vi "PumpValve3.vi"() -> ()   [LabVIEW 2015]
uses:
  PumpValve.ctl
  <vilib>/DAQmx/write.llb/DAQmx Write (Digital 1D Bool NChan 1Samp 1Line).vi
  <vilib>/DAQmx/miscellaneous.llb/DAQmx Fill In Error Info.vi
panel:
  in  "DAQmx Task 3":refnum<k21>
  in  "DAQmx Task 2":refnum<k21>
  in  "DAQmx Task 1":refnum<k21>
  in  "On/Off (Pump)":bool
  in  "Open/Close (Blue)":bool
  in  "Open/Close (Green)":bool
  in  "Manual Mode":bool
  in  "Stop Pumps/Valve":bool
  out "Invalid fill%":bool
  out "Tank":u32(slide) scale=0.0..100.0
  in  "Drain %":u32
  in  "Fill %":u32
  in  "Drain":bool
  in  "Stop Program":bool
  in  "Fill":bool
  out "Green":i32
  out "Blue":i32
  out "Pump":i32
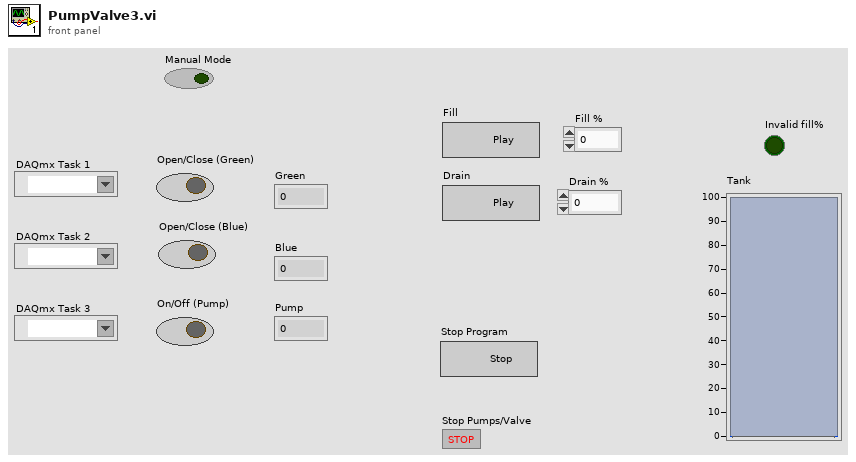
[diagram p1: front panel]
types:
  T1 = typedef "PumpValve.ctl" = enum16{"Manual", "Initialize", "Idle", "Fill", "Drain", "Stop"}
  T2 = cluster{"Open/Close (Green)":bool, "Open/Close (Blue)":bool, "On/Off (Pump)":bool, "off":bool}
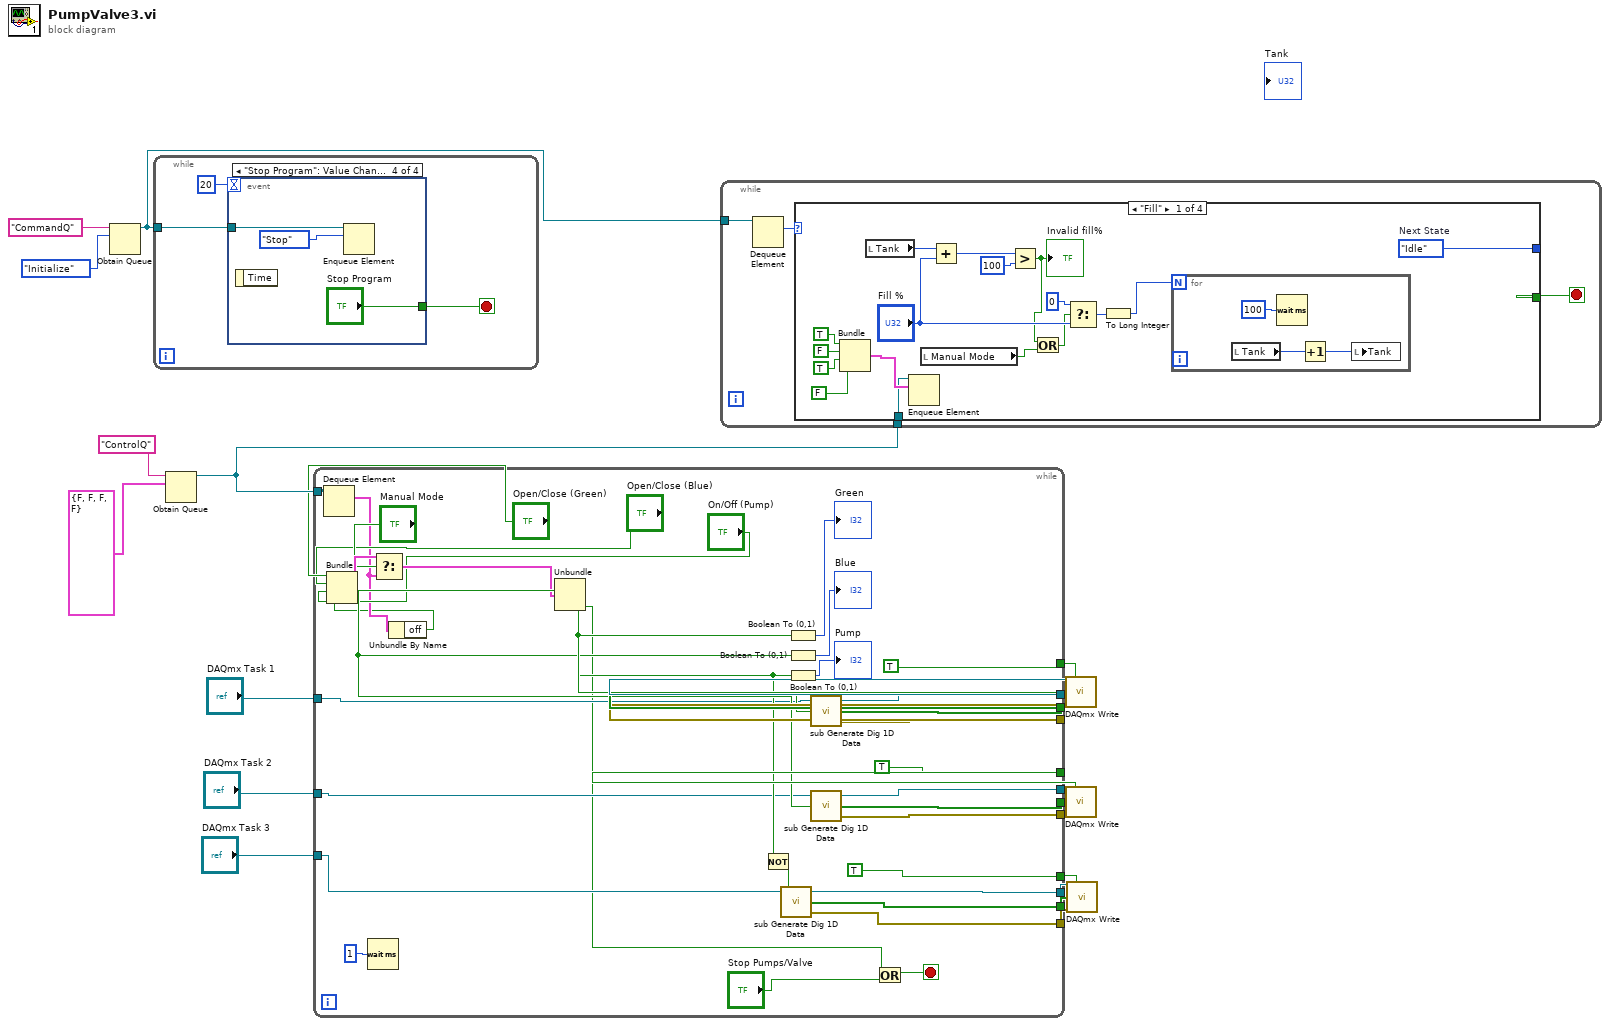
[diagram p0: block diagram]
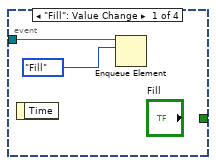
[diagram p2: hidden frame]
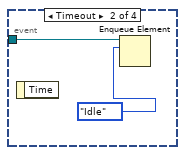
[diagram p3: hidden frame]
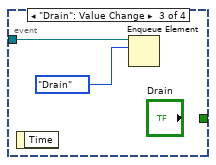
[diagram p4: hidden frame]
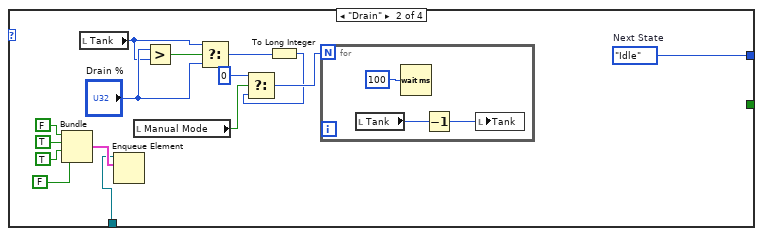
[diagram p5: hidden frame]
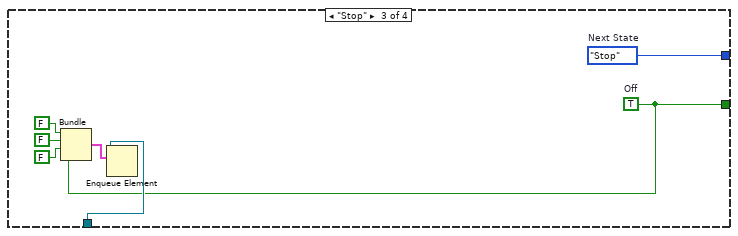
[diagram p6: hidden frame]
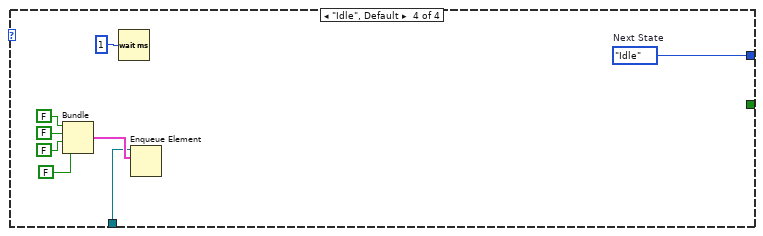
[diagram p7: hidden frame]
diagram:
  n1 = Obtain Queue(name (unnamed)="CommandQ", element data type=PumpValve."Initialize" ("States")) -> (queue out=w20:refnum<queue>)  [unwired: 3 in, 2 out]
  n2 = while {
    tunnel: w20 -> [w22]
    stop <- w23 stop-if-true
    n3 = event shown="[3] \"Stop Program\": Value Change" {
      selector: _ -> [_ _ _ _]
      dyn-events: _ -> [_ _ _ _]
      timeout: 20 -> [_ _ _ _]
      tunnel: [_ _ _ "Stop Program"] -> w23
      tunnel: w22 -> [w26 w28 w30 w33]
      event "Fill": Value Change {
        n4 = event-data() -> ()  [unwired: 1 in, 1 out]
        n5 = Enqueue Element(queue=w26, element=PumpValve."Fill" ("States")) -> ()  [unwired: 2 in, 3 out]
      }
      event Timeout {
        n6 = event-data() -> ()  [unwired: 1 in, 1 out]
        n7 = Enqueue Element(queue=w28, element=PumpValve."Idle" ("States")) -> ()  [unwired: 2 in, 3 out]
      }
      event "Drain": Value Change {
        n8 = event-data() -> ()  [unwired: 1 in, 1 out]
        n9 = Enqueue Element(queue=w30, element=PumpValve."Drain" ("States")) -> ()  [unwired: 2 in, 3 out]
      }
      event "Stop Program": Value Change {
        n10 = event-data() -> ()  [unwired: 1 in, 1 out]
        n11 = Enqueue Element(queue=w33, element=PumpValve."Stop" ("States")) -> ()  [unwired: 2 in, 3 out]
      }
    }
  }
  n12 = Obtain Queue(name (unnamed)="ControlQ", element data type=cluster{bool, bool, bool, "off":bool} {FALSE, FALSE, FALSE, "off"=FALSE}) -> (queue out=w5:refnum<queue>)  [unwired: 3 in, 2 out]
  n13 = while {
    tunnel: w5 -> [w45]
    tunnel: "DAQmx Task 3" -> [w61]
    tunnel: "DAQmx Task 2" -> [w60]
    tunnel: "DAQmx Task 1" -> [w59]
    tunnel: [TRUE] -> w19
    tunnel: [w57] -> w18
    tunnel: [w56] -> w17
    tunnel: [w55] -> w16
    tunnel: [TRUE] -> w15
    tunnel: [w53] -> w14
    tunnel: [w52] -> w13
    tunnel: [w51] -> w12
    tunnel: [TRUE] -> w11
    tunnel: [w49] -> w10
    tunnel: [w48] -> w9
    tunnel: [w47] -> w8
    stop <- w37 stop-if-true
    n14 = Dequeue Element(queue=w45) -> (element=w35:cluster{bool, bool, bool, "off":bool})  [unwired: 2 in, 3 out]
    n15 = Wait (ms)(milliseconds to wait=u32 1) -> ()  [unwired: 1 out]
    n16 = Unbundle By Name(w35) -> ("off"=w34:bool)
    n17 = Bundle("Open/Close (Green)"="Open/Close (Green)", "Open/Close (Blue)"="Open/Close (Blue)", "On/Off (Pump)"="On/Off (Pump)", "off"=w34) -> (w43:T2)  [unwired: 1 in]
    n18 = Select(t=w43, s="Manual Mode", f=w35) -> (s? t:f=w44:T2)
    n19 = Unbundle(w44) -> ("Open/Close (Green)"=w64:bool, "Open/Close (Blue)"=w63:bool, "On/Off (Pump)"=w62:bool, "off"=w38:bool)
    n20 = Not(x=w62) -> (.not. x?=w67:bool)
    n21 = call <vilib>:"sub Generate Dig 1D Data.vi"("initial value"=w67, "task in"=w61) -> ("error out"=w47:errorcluster, "Data"=w48:bool[], "task out"=w49:refnum<k21>)  [unwired: 1 in]
    n22 = Boolean To (0,1)(Boolean=w64) -> (0, 1=→"Green":i16)
    n23 = Boolean To (0,1)(Boolean=w63) -> (0, 1=→"Blue":i16)
    n24 = Boolean To (0,1)(Boolean=w62) -> (0, 1=→"Pump":i16)
    n25 = call <vilib>:"sub Generate Dig 1D Data.vi"("initial value"=w64, "task in"=w59) -> ("error out"=w55:errorcluster, "Data"=w56:bool[], "task out"=w57:refnum<k21>)  [unwired: 1 in]
    n26 = call <vilib>:"sub Generate Dig 1D Data.vi"("initial value"=w63, "task in"=w60) -> ("error out"=w51:errorcluster, "Data"=w52:bool[], "task out"=w53:refnum<k21>)  [unwired: 1 in]
    n27 = Or(x=w38, y="Stop Pumps/Valve") -> (x .or. y?=w37:bool)
  }
  n28 = while {
    tunnel: w20 -> [w72]
    tunnel: w5 -> [w69]
    stop <- w71 stop-if-true
    n29 = Dequeue Element(queue=w72) -> (element=w70:T1)  [unwired: 2 in, 3 out]
    n30 = case shown="\"Fill\"" w70 {
      tunnel: [w89 w107 w117 w125] -> _
      tunnel: [_ _ w111 _] -> w71
      tunnel: w69 -> [w77 w99 w112 w119]
      frame "Fill" {
        w89 = PumpValve."Idle"  # Next State
        n31 = Bundle(TRUE, FALSE, TRUE, FALSE) -> (w78:cluster{bool, bool, bool, bool})  [unwired: 1 in]
        n32 = local read "Tank"() -> (w88:u32)
        n33 = Enqueue Element(queue=w77, element=w78) -> ()  [unwired: 2 in, 3 out]
        n34 = local read "Manual Mode"() -> (w75:bool)
        n35 = Add(x=w88, y="Fill %") -> (x+y=w86:u32)
        n36 = Greater?(x=w86, y=u32 100) -> (0:w76:bool)
        "Invalid fill%" <- w76
        n37 = Or(x=w76, y=w75) -> (x .or. y?=w74:bool)
        n38 = Select(t=u32 0, s=w74, f="Fill %") -> (s? t:f=w83:u32)
        n39 = To Long Integer(number=w83) -> (32bit integer=w82:i32)
        n40 = for {
          N: w82 -> [_]
          n41 = local read "Tank"() -> (w92:u32)
          n42 = Wait (ms)(milliseconds to wait=u32 100 ("y")) -> ()  [unwired: 1 out]
          n43 = Increment(x=w92) -> (x+1=w91:u32)
          n44 = local write "Tank"(w91) -> ()
        }
      }
      frame "Drain" {
        w107 = PumpValve."Idle"  # Next State
        n45 = Bundle(FALSE, TRUE, TRUE, FALSE) -> (w100:cluster{bool, bool, bool, bool})  [unwired: 1 in]
        n46 = local read "Tank"() -> (w104:u32)
        n47 = Enqueue Element(queue=w99, element=w100) -> ()  [unwired: 2 in, 3 out]
        n48 = local read "Manual Mode"() -> (w96:bool)
        n49 = Greater?(x="Drain %", y=w104) -> (0:w97:bool)
        n50 = Select(t=w104, s=w97, f="Drain %") -> (s? t:f=w106:u32)
        n51 = To Long Integer(number=w106) -> (32bit integer=w93:i32)
        n52 = Select(t=0, s=w96, f=w93) -> (s? t:f=w94:i32)
        n53 = for {
          N: w94 -> [_]
          n54 = local read "Tank"() -> (w109:u32)
          n55 = Wait (ms)(milliseconds to wait=u32 100) -> ()  [unwired: 1 out]
          n56 = Decrement(x=w109) -> (x-1=w110:u32)
          n57 = local write "Tank"(w110) -> ()
        }
      }
      frame "Stop" {
        w111 = TRUE  # Off
        w117 = PumpValve."Stop"  # Next State
        n58 = Bundle(FALSE, FALSE, FALSE, "Off"=w111) -> (w113:cluster{bool, bool, bool, "Off":bool})  [unwired: 1 in]
        n59 = Enqueue Element(queue=w112, element=w113) -> ()  [unwired: 2 in, 3 out]
      }
      frame "Idle", Default {
        w125 = PumpValve."Idle"  # Next State
        n60 = Bundle(FALSE, FALSE, FALSE, FALSE) -> (w120:cluster{bool, bool, bool, bool})  [unwired: 1 in]
        n61 = Wait (ms)(milliseconds to wait=u32 1) -> ()  [unwired: 1 out]
        n62 = Enqueue Element(queue=w119, element=w120) -> ()  [unwired: 2 in, 3 out]
      }
    }
  }
  n63 = call-poly <vilib>:"DAQmx Write.vi"("task/channels in"=w18, "auto start"=w19, "data"=w17, "error in"=w16) -> ()  [unwired: 9 in, 3 out]
  n64 = call-poly <vilib>:"DAQmx Write.vi"("task/channels in"=w14, "auto start"=w15, "data"=w13, "error in"=w12) -> ()  [unwired: 9 in, 3 out]
  n65 = call-poly <vilib>:"DAQmx Write.vi"("task/channels in"=w10, "auto start"=w11, "data"=w9, "error in"=w8) -> ()  [unwired: 9 in, 3 out]
